vi "Request-Response Example.vi"   [LabVIEW 2024]
uses:
  NATS Infrastructure/NATS Infrastructure.lvlib
panel:
  # "Instructions:\n\n0. Install NATS-Server. If not installed, run Server Install.vi\nSee the diagram disable strcture on the block diagram \nfor more details.\n1. Run this VI\n2. Update the Subject Payload in Requester.vi\n3. Watch for an updated response from Responder.vi"
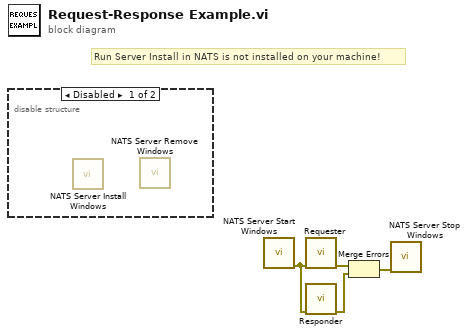
[diagram p0: block diagram]
diagram:
  # "Run Server Install in NATS is not installed on your machine!"
  n1 = disable-structure shown="Disabled" {
    frame Disabled {
      n2 = call "NATS Server Install Windows.vi"() -> ()  [unwired: 11 in, 1 out]
      n3 = call "NATS Server Remove Windows.vi"() -> ()  [unwired: 11 in, 1 out]
    }
    frame Enabled {
    }
  }
  n4 = call "NATS Server Start Windows.vi"() -> ("error out"=w3:errorcluster)  [unwired: 11 in]
  n5 = call "Requester.vi"("error in"=w3) -> ("error out"=w1:errorcluster)  [unwired: 10 in]
  n6 = call "Responder.vi"("error in"=w3) -> ("error out"=w4:errorcluster)  [unwired: 10 in]
  n7 = Merge Errors(w1, w4) -> (w2:errorcluster)
  n8 = call "NATS Server Stop Windows.vi"("error in"=w2) -> ()  [unwired: 10 in, 1 out]
